vi "Enforce Limits.vi"(6 "Device":string, 7 "Setpoint":dbl, 8 "error in":errorcluster, 9 "Minimum":dbl, 10 "Maximum":dbl, 11 "Previous":dbl) -> (0 "error out":errorcluster, 2 "Protected Setpoint":dbl)   [LabVIEW 2023, in "Instruments.lvlib" / "Instruments.lvclass"]
uses:
  Library/Instruments.lvclass
  <vilib>/Utility/error.llb/Error Cluster From Error Code.vi
  <vilib>/ErrorRing/Error Ring.xnode
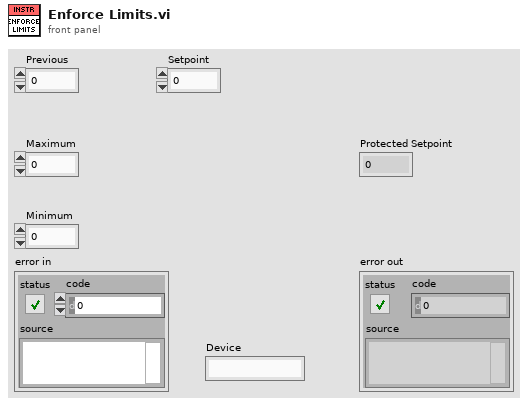
[diagram p1: front panel]
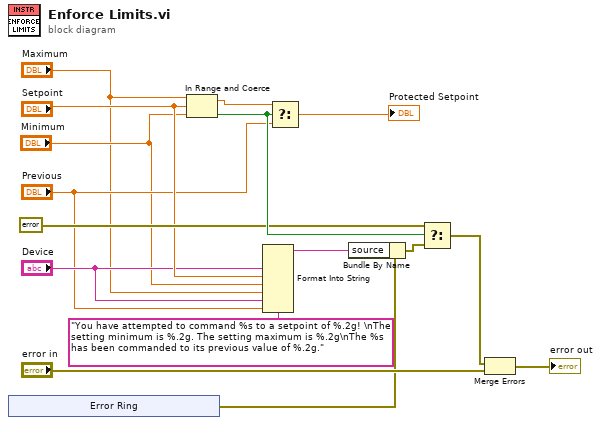
[diagram p0: block diagram]
diagram:
  n1 = xnode "Error Ring"() -> ("error out"=w11:errorcluster)
  n2 = In Range and Coerce(upper limit="Maximum", x="Setpoint", lower limit="Minimum") -> (coerced(x)=w9:dbl, In Range?=w16:bool)
  n3 = Format Into String(format string="You have attempted to command %s to a setpoint of %.2g! \nThe setting minimum is %.2g. The setting maximum is %.2g\nThe %s has been commanded to its previous value of %.2g.", "Device", "Setpoint", "Minimum", "Maximum", "Device", "Previous") -> (resulting string=w7:string)  [unwired: 2 in, 1 out]
  n4 = Select(t=w9, s=w16, f="Previous") -> (s? t:f=→"Protected Setpoint":dbl)
  n5 = Bundle By Name(cluster=w11, "source"=w7) -> (w8:errorcluster)
  n6 = Select(t=errorcluster {"status"=FALSE, "code"=0, "source"=""}, s=w16, f=w8) -> (s? t:f=w13:errorcluster)
  n7 = Merge Errors(w13, "error in") -> (→"error out":errorcluster)
